vi "ILABW_CreateFromTemplate.vi"(3 "path":string, 4 "suffix":string, 5 "templateName":string) -> (0 "VI Path":path, 1 "name":string)   [LabVIEW 2012]
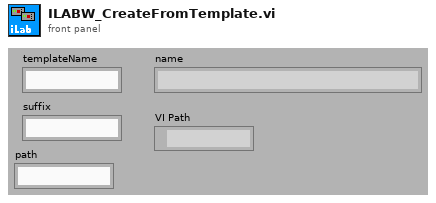
[diagram p1: front panel]
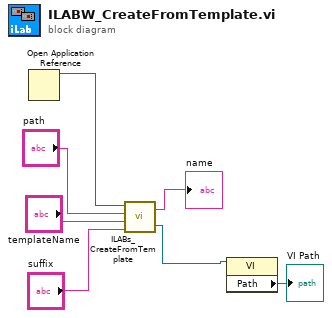
[diagram p0: block diagram]
diagram:
  n1 = Open Application Reference() -> (3:w7:refnum<vi>)  [unwired: 1 in, 4 out]
  n2 = call "ILABs_CreateFromTemplate.vi"("suffix"="suffix", "templateName"="templateName", "path"="path", "appRef"=w7) -> ("viReference"=w2:refnum<vi>, "name"=→"name":string)
  n3 = property class="VI"(reference=w2) -> ("Path"=→"VI Path":path)  [unwired: 1 in, 2 out]
